vi "LinxSpiConfigure.vi"(8 "Error In":errorcluster, 9 "SPI Configuration":T1={"Clock Frequency"=1000000, "Bit Order"=enum."LSb First", "SPI Mode"=enum."Mode 0"}, 10 "SPI Channel":u8, 11 "LINX Resource":T4) -> (0 "Error Out":errorcluster, 2 "actualSpeed":u32, 3 "LINX Resource":T4)   [LabVIEW 2020, in "LMH-LINX.lvlib" / "Local IO.lvlib"]
uses:
  Local IO.lvlib
  Type Defs/LINX Ref.ctl
  Type Defs/Platform.ctl
  Type Defs/Interface.ctl
  Device/Type Defs/LINX Device Config.ctl
  Device/Type Defs/TCP Config.ctl
  Device/Type Defs/Channels.ctl
  Type Defs/Peripherals/SPI/SPI Configuration.ctl
  Type Defs/Peripherals/SPI/SPI Bit Order.ctl
  Type Defs/Peripherals/SPI/SPI Mode.ctl
  Type Defs/Error Type.ctl
  LMH-LINX.lvlib
  <vilib>/MakerHub/LINX/Resources/liblinxdevice.dll
  Device/Device.lvlib
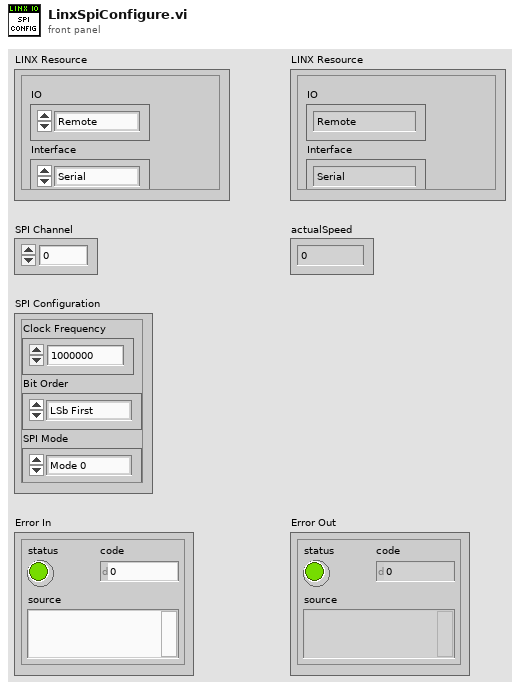
[diagram p1: front panel]
types:
  T1 = typedef "LMH-LINX.lvlib/SPI Configuration.ctl" = cluster{"Clock Frequency":u32, "Bit Order":T2, "SPI Mode":T3}
  T2 = typedef "LMH-LINX.lvlib/SPI Bit Order.ctl" = enum8{"LSb First", "MSb First"}
  T3 = typedef "LMH-LINX.lvlib/SPI Mode.ctl" = enum8{"Mode 0", "Mode 1", "Mode 2", "Mode 3"}
  T4 = typedef "LMH-LINX.lvlib/LINX Ref.ctl" = cluster{"IO":T5, "Interface":T6, "LINX Device Config":T7}
  T5 = typedef "LMH-LINX.lvlib/Platform.ctl" = enum16{"Remote", "Local"}
  T6 = typedef "LMH-LINX.lvlib/Interface.ctl" = enum16{"Serial", "TCP"}
  T7 = typedef "LMH-LINX.lvlib/Device.lvlib/LINX Device Config.ctl" = cluster{"Interface":T6, "COM Port":refnum<visa-resource-name>, "TCP Configuration":T8, "Device Family":u8, "Device ID":u8, "Device Name":string, "TCP Ref":refnum<k5>, "Channels":T9}
  T8 = typedef "LMH-LINX.lvlib/Device.lvlib/TCP Config.ctl" = cluster{"IP Address":string, "Port":u16}
  T9 = typedef "LMH-LINX.lvlib/Channels.ctl" = cluster{"DI":u8[], "DO":u8[], "AI":u8[], "AO":u8[], "PWM":u8[], "QE":u8[], "UART":u8[], "I2C 2":u8[], "SPI":u8[], "CAN":u8[], "Servo":u8[], "AI Ref (V)":dbl, "AI Resolution (Bits)":u8, "AO Ref (V)":dbl, "AO Resolution (Bits)":u8}
  T10 = typedef "LMH-LINX.lvlib/Error Type.ctl" = enum16{"Unknown", "Timeout", "Corrupt Return Packet", "Unable To Connect", "Command Not Supported", "Channel DNE", "Invalid COM Config", "Firmware Version Mismatch", "myRIO Support", "CMD Specific Error", "Local IO Not Supported"}
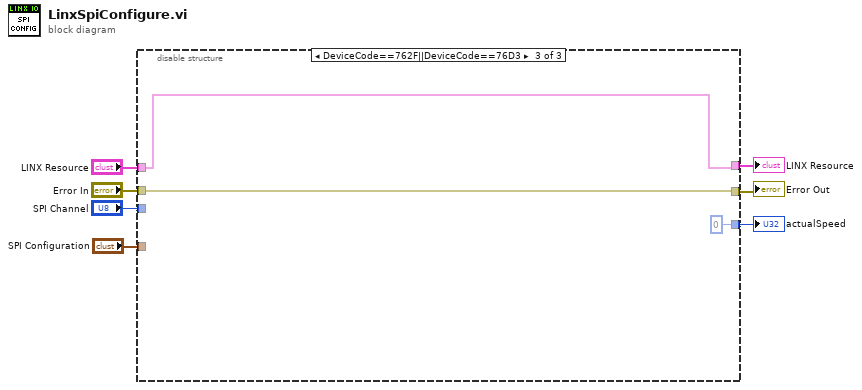
[diagram p0: block diagram]
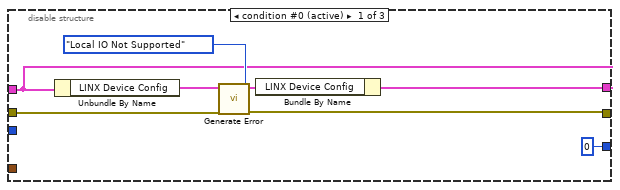
[diagram p2: hidden frame]
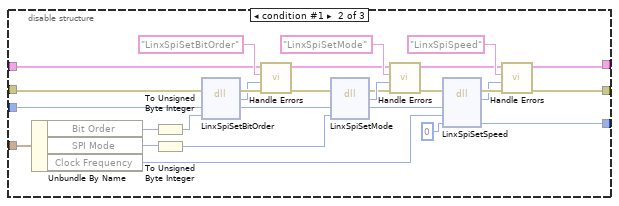
[diagram p3: hidden frame]
diagram:
  n1 = disable-structure shown="DeviceCode==762F||DeviceCode==76D3" {
    disable-tunnel: [w10 w17 w45] -> w7
    disable-tunnel: "LINX Resource" -> [w12 w38 w45]
    disable-tunnel: "Error In" -> [w14 w41 w46]
    disable-tunnel: "SPI Channel" -> [_ w39 _]
    disable-tunnel: "SPI Configuration" -> [_ w37 _]
    disable-tunnel: [u32 0 ("actualSpeed") w18 u32 0 ("actualSpeed")] -> w2
    disable-tunnel: [w8 w16 w46] -> w1
    frame condition #0 (active) {
      n2 = Unbundle By Name(w12) -> ("LINX Device Config"=w13:T7)
      n3 = call "Generate Error.vi"("Error In"=w14, "Error Type"=Error_Type."Local IO Not Supported", "LINX Device Config"=w13) -> ("Error Out"=w8:errorcluster, "Dup LINX Device Config"=w11:T7)  [unwired: 7 in]
      n4 = Bundle By Name(cluster=w12, "LINX Device Config"=w11) -> (w10:T4)
    }
    frame condition #1 {
      n5 = Unbundle By Name(w37) -> ("Bit Order"=w36:T2, "SPI Mode"=w28:T3, "Clock Frequency"=w20:u32)
      n6 = To Unsigned Byte Integer(number=w36) -> (unsigned 8bit integer=w35:u8)
      n7 = To Unsigned Byte Integer(number=w28) -> (unsigned 8bit integer=w27:u8)
      n8 = dll-call lib="C:/Program Files (x86)/National Instruments/LabVIEW 2020/vi.lib/MakerHub/LINX/Resources/liblinxdevice.*" fn="LinxSpiSetBitOrder"(error in=w41, "channel"=w39, "bitOrder"=w35) -> (error out=w42:errorcluster, "Status"=w40:i32, "channel"=w29:u8)  [unwired: 3 in, 1 out]
      n9 = call <vilib>:"Handle Errors.vi"("Error In"=w42, "LinxStatus"=w40, "Function Name"="LinxSpiSetBitOrder", "LINX Resource"=w38) -> ("Error Out"=w31:errorcluster, "LINX Resource"=w30:T4)  [unwired: 6 in]
      n10 = dll-call lib="C:/Program Files (x86)/National Instruments/LabVIEW 2020/vi.lib/MakerHub/LINX/Resources/liblinxdevice.*" fn="LinxSpiSetMode"(error in=w31, "channel"=w29, "mode"=w27) -> (error out=w33:errorcluster, "Status"=w34:i32, "channel"=w21:u8)  [unwired: 3 in, 1 out]
      n11 = call <vilib>:"Handle Errors.vi"("Error In"=w33, "LinxStatus"=w34, "Function Name"="LinxSpiSetMode", "LINX Resource"=w30) -> ("Error Out"=w23:errorcluster, "LINX Resource"=w22:T4)  [unwired: 6 in]
      n12 = dll-call lib="C:/Program Files (x86)/National Instruments/LabVIEW 2020/vi.lib/MakerHub/LINX/Resources/liblinxdevice.*" fn="LinxSpiSetSpeed"(error in=w23, "channel"=w21, "speed"=w20, "actualSpeed"=u32 0) -> (error out=w25:errorcluster, "Status"=w24:i32, "actualSpeed"=w18:u32)  [unwired: 4 in, 1 out]
      n13 = call <vilib>:"Handle Errors.vi"("Error In"=w25, "LinxStatus"=w24, "Function Name"="LinxSpiSpeed", "LINX Resource"=w22) -> ("Error Out"=w16:errorcluster, "LINX Resource"=w17:T4)  [unwired: 6 in]
    }
    frame condition #2 {
    }
  }
  "LINX Resource" <- w7
  "Error Out" <- w1
  "actualSpeed" <- w2
